vi "Begin.vi"() -> (0 "error out":errorcluster)   [LabVIEW 2012]
doc: "Called before other user functions, this VI is expected to open initial I/O refnums, load in file data, and do all program initialization. Notice that the <B>error out</B> terminal is simply used for data flow. Wiring it to other structures or subVIs ensures that this VI runs first."
uses:
  <vilib>/Rock Robotics/WPI/SafetyOutput/WPI_SafetyOutputConfigMenu.ctl
  <vilib>/Rock Robotics/WPI/DriverStation/WPI_DriverStationRobotMode2.ctl
  <vilib>/Rock Robotics/WPI/Joystick/WPI_JoystickDeviceEnum.ctl
  <vilib>/Rock Robotics/WPI/CAN/Jaguar/SubVIs/WPI_CANJaguar_BrakeCoastMode.ctl
  Robot Global Data.vi
  <vilib>/Rock Robotics/WPI/RobotDrive/WPI_RobotDriveOpen4MotorWithExistingMotors.vi
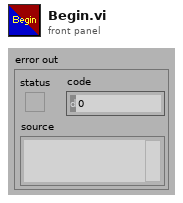
[diagram p1: front panel]
types:
  T1 = typedef "WPI_CANJaguar_BrakeCoastMode.ctl" = enum8{"Jumper", "Brake", "Coast"}
  T2 = typedef "WPI_JoystickDeviceEnum.ctl" = enum16{"USB 1", "USB 2", "USB 3", "USB 4", "Kinect 1", "Kinect 2"}
  T3 = typedef "WPI_DriverStationRobotMode2.ctl" = enum16{"Autonomous Disabled", "Autonomous Enabled", "Teleop Disabled", "Teleop Enabled", "Timeout", "Finish", "Test Disabled", "Test Enabled"}
  T4 = typedef "WPI_SafetyOutputConfigMenu.ctl" = enum16{"Enable", "Disable"}
  T5 = typedef "WPI_MotorControlDeviceRef.ctl" = cluster{"DeviceStatus":errorcluster, "Type":enum16{"PWM", "CAN"}, "PWM":cluster{"Digital Module":T6, "PWM Channel":T7, "DeadBand":T8}, "CAN":cluster{"Device Number":u8, "Control Mode":T9, "Semaphore":T10, "Max Vout":dbl}, "Invert":bool, "TransformRef":T11, "InvTransformRef":T11}
  T6 = typedef "FPGA_TypedefDigitalModule.ctl" = enum16{"Digital Module 1", "Digital Module 2"}
  T7 = typedef "FPGA_DIOPWMChannel.ctl" = enum8{"PWM 1", "PWM 2", "PWM 3", "PWM 4", "PWM 5", "PWM 6", "PWM 7", "PWM 8", "PWM 9", "PWM 10", "Invalid"}
  T8 = typedef "WPI_PWMDeadband.ctl" = cluster{"Name":string, "maxPositivePwm":i32, "minPositivePwm":i32, "centerPwm":i32, "maxNegativePwm":i32, "minNegativePwm":i32, "angularRange":u16}
  T9 = typedef "WPI_CANJaguar_ControlMode.ctl" = enum8{"Percent VBus", "Current", "Speed", "Position", "Voltage"}
  T10 = typedef "Semaphore RefNum" = refnum<k1>
  T11 = typedef "WPI_PWMTransform_ConPane.ctl" = refnum<vi>
  T12 = typedef "WPI_JoystickDevRef.ctl" = cluster{"Device":T2}
  T13 = typedef "WPI_RobotDriveDevRef.ctl" = cluster{"DevStatus":errorcluster, "Motors[]":T5[], "Square Inputs":bool, "Max Output":dbl, "Isochronous":bool}
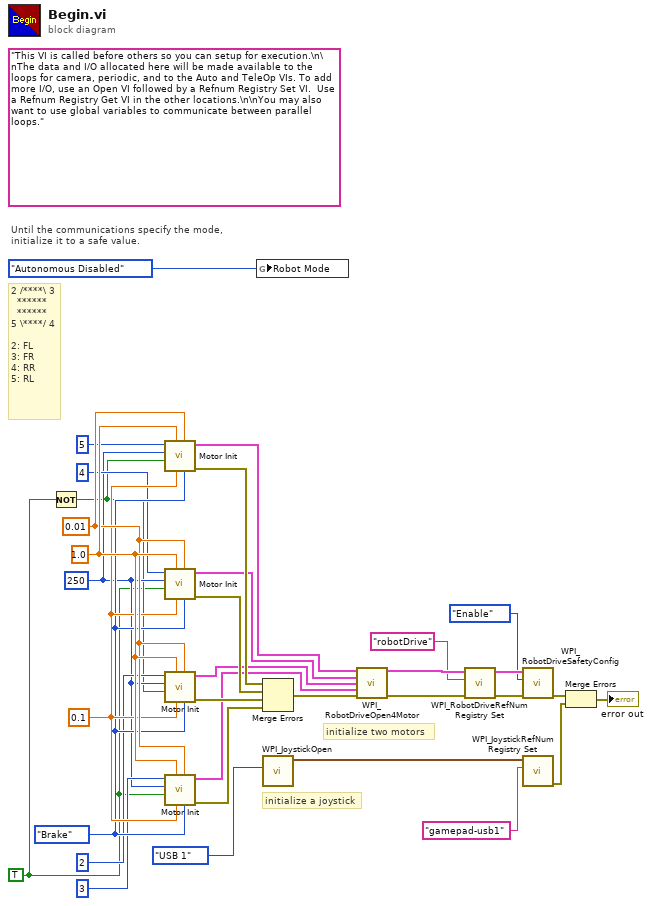
[diagram p0: block diagram]
diagram:
  w1 = TRUE ("x")
  w3 = u16 250 ("Encoder Codes Per Rev")
  w16 = WPI_CANJaguar_BrakeCoastMode."Brake" ("Brake / Coast Mode")
  w21 = 0.1 ("D")
  w22 = 0.01 ("I")
  w23 = 1.0 ("P")
  (unwired) "This VI is called before others so you can setup for execution.\n\nThe data and I/O allocated here will be made available to the loops for camera, periodic, and to the Auto and TeleOp VIs. To add more I/O, use an Open VI followed by a Refnum Registry Set VI.  Use a Refnum Registry Get VI in the other locations.\n\nYou may also want to use global variables to communicate between parallel loops."
  # "2 /****\\ 3\n  ******\n  ******\n5 \\****/ 4\n\n2: FL\n3: FR\n4: RR\n5: RL"
  # "initialize a joystick"
  # "Until the communications specify the mode,\ninitialize it to a safe value."
  # "initialize two motors"
  n1 = Not(x=w1) -> (.not. x?=w2:bool)
  n2 = call "Motor Init.vi"("Brake / Coast Mode"=w16, "I"=w22, "D"=w21, "P"=w23, "Invert"=w2, "Encoder Codes Per Rev"=w3, "Device Number"=u8 5) -> ("error out"=w20:errorcluster, "CAN Jaguar Ref Out"=w11:T5)  [unwired: 3 in]
  n3 = call "Motor Init.vi"("Brake / Coast Mode"=w16, "I"=w22, "D"=w21, "P"=w23, "Invert"=w1, "Encoder Codes Per Rev"=w3, "Device Number"=u8 4) -> ("error out"=w19:errorcluster, "CAN Jaguar Ref Out"=w10:T5)  [unwired: 3 in]
  n4 = call "Motor Init.vi"("Brake / Coast Mode"=w16, "I"=w22, "D"=w21, "P"=w23, "Invert"=w2, "Encoder Codes Per Rev"=w3, "Device Number"=u8 2) -> ("error out"=w18:errorcluster, "CAN Jaguar Ref Out"=w9:T5)  [unwired: 3 in]
  n5 = call "Motor Init.vi"("Brake / Coast Mode"=w16, "I"=w22, "D"=w21, "P"=w23, "Invert"=w1, "Encoder Codes Per Rev"=w3, "Device Number"=u8 3) -> ("error out"=w17:errorcluster, "CAN Jaguar Ref Out"=w8:T5)  [unwired: 3 in]
  n6 = global write "Robot Global Data.vi" "Robot Mode"(WPI_DriverStationRobotMode2."Autonomous Disabled" ("Robot Mode")) -> ()
  n7 = Merge Errors(w20, w19, w18, w17) -> (w15:errorcluster)
  n8 = call <vilib>:"WPI_JoystickOpen.vi"("JoystickDevice"=WPI_JoystickDeviceEnum."USB 1") -> ("JoystickDevRef"=w26:T12)  [unwired: 10 in]
  n9 = call-poly <vilib>:"WPI_RobotDriveOpen4Motor.vi"("Rear Left Motor Dev Ref"=w11, "Rear Right Motor Dev Ref"=w10, "Front Left Motor Dev Ref"=w9, "Front Right Motor Dev Ref"=w8, "error in (no error)"=w15) -> ("RobotDriveDevRef"=w33:T13, "error out"=w31:errorcluster)  [unwired: 9 in]
  n10 = call <vilib>:"WPI_RobotDriveRefNum Registry Set.vi"("error in (no error)"=w31, "refnum name"="robotDrive", "RobotDriveDevRef"=w33) -> ("error out"=w14:errorcluster, "RobotDriveDevRef"=w30:T13)  [unwired: 7 out]
  n11 = call <vilib>:"WPI_RobotDriveSafetyConfig.vi"("error in (no error)"=w14, "mode"=WPI_SafetyOutputConfigMenu."Enable", "RobotDriveDevRef"=w30) -> ("error out"=w13:errorcluster)  [unwired: 7 in, 1 out]
  n12 = call <vilib>:"WPI_JoystickRefNum Registry Set.vi"("refnum name"="gamepad-usb1", "JoystickDevRef"=w26) -> ("error out"=w12:errorcluster)  [unwired: 8 in, 1 out]
  n13 = Merge Errors(w13, w12) -> (→"error out":errorcluster)
